vi "Reserve GPIO.vi"(8 "error in (no error)":errorcluster, 9 "Purpose":string, 10 "GPIO #":T1=-1, 11 "Session in":refnum<class "Session.lvclass">) -> (0 "error out":errorcluster, 3 "Session out":refnum<class "Session.lvclass">)   [LabVIEW 2020, in "CTI.lvlib" / "Session.lvclass"]
uses:
  Session.lvclass
  Session.lvclass/Session.ctl
  Resource/Resource.lvclass
  b0dc19c6-2fe7-4db4-b436-acd347f0001e.vi
  3105c3fa-af8c-4e6e-a6e2-f897f365ae97.vi
  GPIO/GPIO.lvclass
  C:/dev/cti/cti-drivers-lv-visa/CTI/Resource/Resource.lvclass
  C:/dev/cti/cti-drivers-lv-visa/CTI/GPIO/GPIO.lvclass
  GPIO Number.ctl
  CTI.lvlib
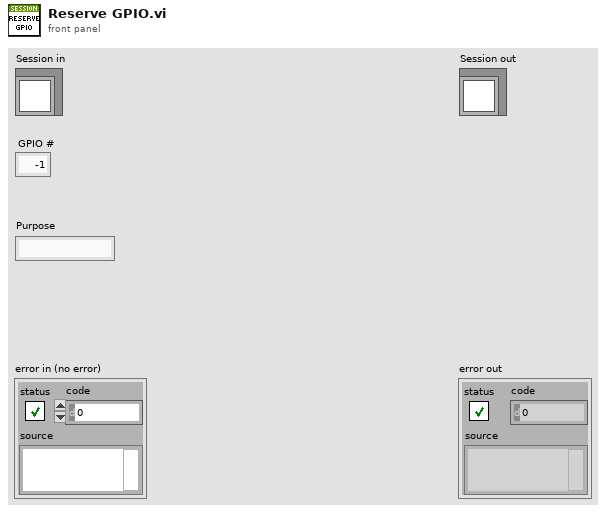
[diagram p1: front panel]
types:
  T1 = typedef "CTI.lvlib/GPIO Number.ctl" = i8
  T2 = typedef "CTI.lvlib/Session.lvclass/Resources.ctl" = cluster{"GPIO":map{T1, refnum<class "GPIO.lvclass">}, "AI":map{T3, refnum<class "AI.lvclass">}, "PWM":map{T1, refnum<class "PWM.lvclass">}, "UART":map{T4, refnum<class "UART.lvclass">}, "I2C":map{T5, refnum<class "I2C.lvclass">}, "SPI":map{T6, refnum<class "SPI.lvclass">}, "SPI CS":map{T1, refnum<class "SPI CS.lvclass">}}
  T3 = typedef "CTI.lvlib/ADC Number.ctl" = i8
  T4 = typedef "CTI.lvlib/UART Number.ctl" = i8
  T5 = typedef "CTI.lvlib/I2C Number.ctl" = i8
  T6 = typedef "CTI.lvlib/SPI Number.ctl" = i8
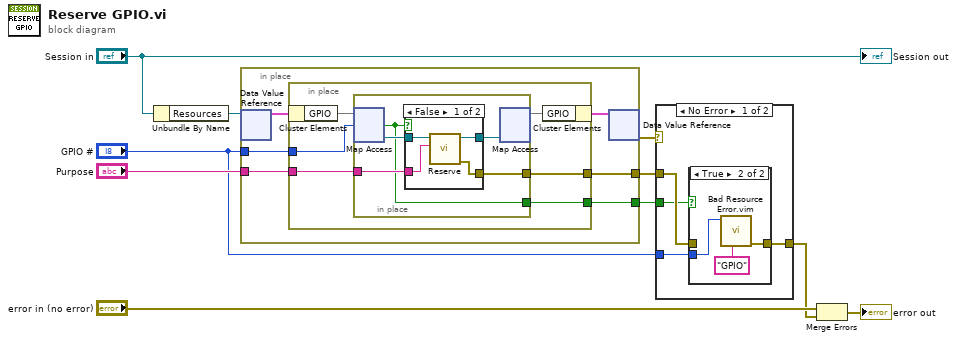
[diagram p0: block diagram]
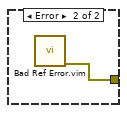
[diagram p3: hidden frame]
diagram:
  n1 = Unbundle By Name("Session in") -> ("Resources"=w10:refnum<data-value>)
  n2 = in-place {
    in-place-border: "GPIO #" -> [w16]
    in-place-border: "Purpose" -> [w15]
    in-place-border: [w14] -> w4
    in-place-border: [w13] -> w7
    n3 = in-place-dvr #1(w10) -> (w11:T2)  [unwired: 1 out]
    n4 = in-place {
      in-place-border: w16 -> [w21]
      in-place-border: w15 -> [w20]
      in-place-border: [w19] -> w14
      in-place-border: [w18] -> w13
      n5 = in-place-cluster #2(w11) -> ("GPIO"=w22:map{T1, refnum<class "GPIO.lvclass">})
      n6 = in-place {
        in-place-border: w20 -> [w26]
        in-place-border: [w25] -> w18
        in-place-border: [w24] -> w19
        n7 = in-place-map #3(w22, w21) -> (w27:refnum<class "GPIO.lvclass">, w24:bool)  [unwired: 1 in]
        n8 = case shown="False" w24 {
          tunnel: w27 -> [w31 w32]
          tunnel: w26 -> [w30 _]
          tunnel: [w29 w32] -> w23
          tunnel: [w28 _] -> w25
          frame False {
            n9 = call "Reserve.vi"("Purpose"=w30, "Resource in"=w31) -> ("error out"=w28:errorcluster, "Resource out"=w29:refnum<class "GPIO.lvclass">)  [unwired: 8 in]
          }
          frame True {
          }
        }
        n10 = in-place-map #3(w23) -> (w17:map{T1, refnum<class "GPIO.lvclass">})  [unwired: 1 in, 2 out]
      }
      n11 = in-place-cluster #2("GPIO"=w17) -> (w12:T2)
    }
    n12 = in-place-dvr #1(w12) -> (w6:errorcluster)  [unwired: 1 out]
  }
  n13 = case shown="No Error" w6 {
    tunnel: w7 -> [w36 _]
    tunnel: w4 -> [w35 _]
    tunnel: [w34 w41] -> w1
    tunnel: "GPIO #" -> [w33 _]
    frame No Error {
      n14 = case shown="True" w35 {
        tunnel: w36 -> [w37 _]
        tunnel: [w37 w40] -> w34
        tunnel: w33 -> [_ w39]
        frame False {
        }
        frame True {
          n15 = call "Bad Resource Error.vim"("Resource Type"="GPIO", "Res #"=w39) -> ("error out"=w40:errorcluster)  [unwired: 9 in]
        }
      }
    }
    frame Error {
      n16 = call "Bad Ref Error.vim"() -> ("error out"=w41:errorcluster)  [unwired: 10 in, 1 out]
    }
  }
  n17 = Merge Errors("error in (no error)", w1) -> (→"error out":errorcluster)
  "Session out" <- "Session in"
